vi "Get Offset.vi"(8 "error in (no error)":errorcluster, 11 "Domino Laser module Class in":refnum<class "Domino Laser module Class.lvclass">) -> (0 "error out":errorcluster, 1 "Y offset":string, 2 "X offset":string, 3 "Domino Laser module Class out":refnum<class "Domino Laser module Class.lvclass">)   [LabVIEW 2024, in "Domino LM.lvlib" / "Domino Laser module Class.lvclass"]
uses:
  CTRLS/Domino Laser module Class.lvclass
  <vilib>/Utility/error.llb/Trim Whitespace One-Sided.vi
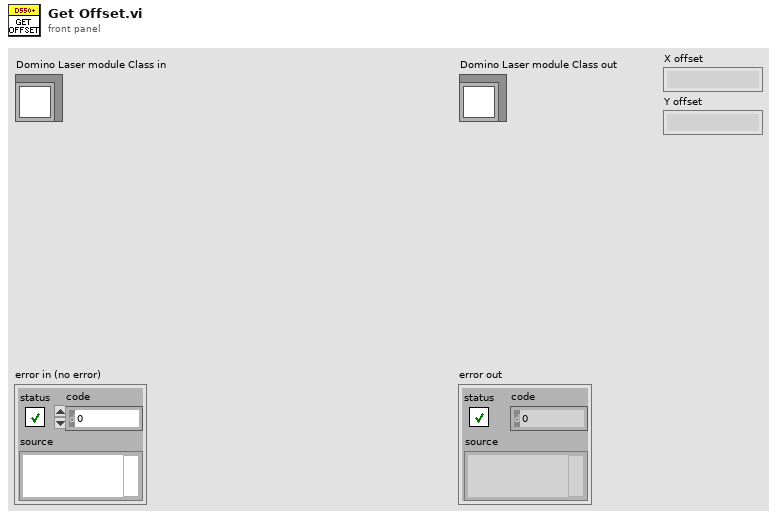
[diagram p1: front panel]
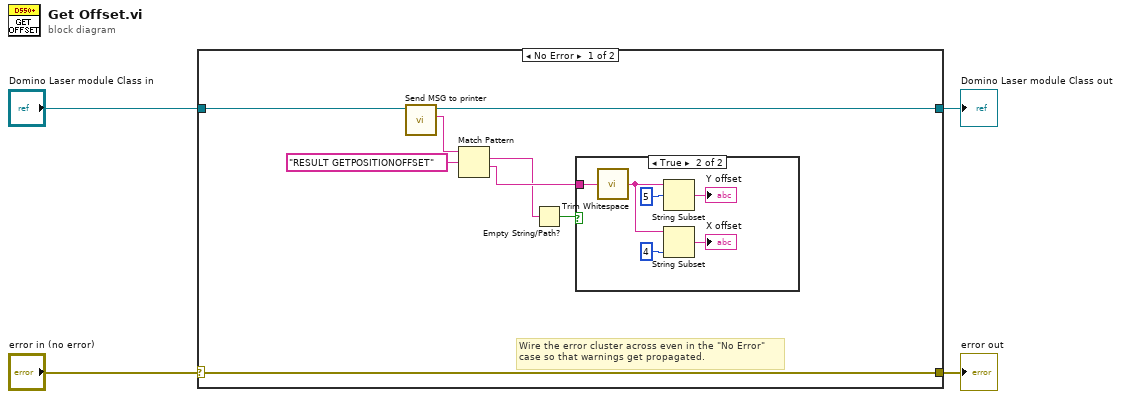
[diagram p0: block diagram]
diagram:
  n1 = case shown="No Error" "error in (no error)" {
    selector: "error in (no error)" -> [w12 w20]
    tunnel: [w12 w20] -> w3
    tunnel: [w10 w19] -> w1
    tunnel: "Domino Laser module Class in" -> [w11 w19]
    frame No Error {
      # "Wire the error cluster across even in the \"No Error\"\ncase so that warnings get propagated."
      n2 = call "Send MSG to printer.vi"("Domino Laser module Class in"=w11) -> ("Recived message"=w9:string, "Domino Laser module Class out"=w10:refnum<class "Domino Laser module Class.lvclass">)  [unwired: 8 in, 1 out]
      n3 = Match Pattern(string=w9, regular expression="RESULT GETPOSITIONOFFSET") -> (match substring=w5:string, after substring=w7:string)  [unwired: 1 in, 2 out]
      n4 = Empty String/Path?(string/path=w5) -> (empty?=w6:bool)
      n5 = case shown="True" w6 {
        tunnel: w7 -> [_ w15]
        frame False {
        }
        frame True {
          n6 = call <vilib>:"Trim Whitespace.vi"("string"=w15) -> ("trimmed string"=w17:string)  [unwired: 1 in]
          n7 = String Subset(string=w17, offset (0)=5) -> (substring=→"Y offset":string)  [unwired: 1 in]
          n8 = String Subset(string=w17, length (rest)=4 ("length (rest)")) -> (substring=→"X offset":string)  [unwired: 1 in]
        }
      }
    }
    frame Error {
    }
  }
  "error out" <- w3
  "Domino Laser module Class out" <- w1
